vi "validate.vi"(8 "error in":errorcluster, 11 "configuration in":refnum<class "PL_Target Configuration.lvclass">) -> (0 "error out":errorcluster, 3 "configuration out":refnum<class "PL_Target Configuration.lvclass">)   [LabVIEW 2013, in "PL_Target Configuration.lvclass"]
doc: "Provides an interface for performing validation on a given configuration. Any children should define the behavior of this function to ensure that the configuration in memory can be used by the runtime class."
uses:
  PL_Target Configuration.lvclass
  <vilib>/NI/Tag Bus Module Framework/root configuration/TBM configuration.lvclass
  PL_Target Configuration.lvclass/PL_Target Configuration.ctl
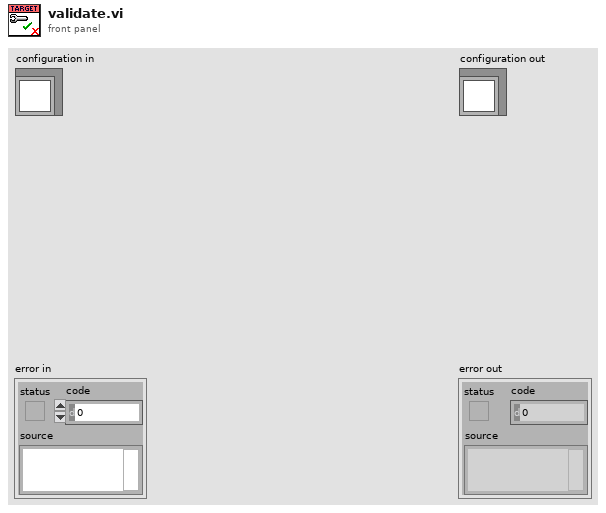
[diagram p1: front panel]
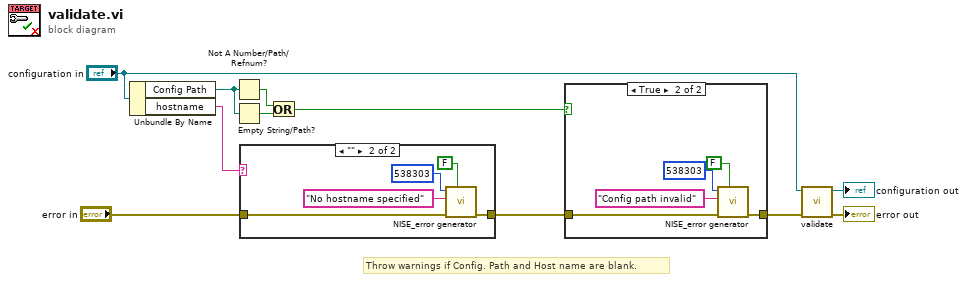
[diagram p0: block diagram]
diagram:
  # "Throw warnings if Config. Path and Host name are blank."
  n1 = Unbundle By Name("configuration in") -> ("Config Path"=w4:path, "hostname"=w1:string)
  n2 = Not A Number/Path/Refnum?(number/path/refnum=w4) -> (NaN/Path/Refnum?=w7:bool)
  n3 = Empty String/Path?(string/path=w4) -> (empty?=w8:bool)
  n4 = case shown="\"\"" w1 {
    tunnel: [w12 w16] -> w3
    tunnel: "error in" -> [w12 w17]
    frame Default {
    }
    frame "" {
      n5 = call <vilib>:"NISE_error generator.vi"("error (T)"=FALSE, "error in"=w17, "append error message"="No hostname specified" ("error message (\"\")"), "error code (0)"=538303) -> ("error out"=w16:errorcluster)  [unwired: 5 in]
    }
  }
  n6 = Or(x=w7, y=w8) -> (x .or. y?=w6:bool)
  n7 = case shown="True" w6 {
    tunnel: [w18 w21] -> w5
    tunnel: w3 -> [w18 w22]
    frame False {
    }
    frame True {
      n8 = call <vilib>:"NISE_error generator.vi"("error (T)"=FALSE, "error in"=w22, "append error message"="Config path invalid" ("error message (\"\")"), "error code (0)"=538303) -> ("error out"=w21:errorcluster)  [unwired: 5 in]
    }
  }
  n9 = call-parent "validate.vi"("error in"=w5, "configuration in"="configuration in") -> ("error out"=→"error out":errorcluster, "configuration out"=→"configuration out":refnum<class "PL_Target Configuration.lvclass">)  [unwired: 8 in]
